vi "Experiment header-Save_Load mov cor section.vi"(7 "Input Mode (ref)":enum16{"Use reference", "Use folder path"}(ring), 8 "error in (no error)":errorcluster, 9 "Function":enum16{"Write", "Read"}(ring), 10 "Experiment folder path":path, 11 "Exp header file ref in":T1) -> (0 "error out":errorcluster, 2 "MovCor enabled (value from header file)":bool, 3 "Exp header file ref":T1)   [LabVIEW 2017]
uses:
  <vilib>/Utility/config.llb/Config Data RefNum.ctl
  Global Variables/General Globals.vi
  <vilib>/Utility/config.llb/Read Key (Boolean).vi
  Movement Correction/Globals/gl_Movement correction globals.vi
  <vilib>/Utility/config.llb/Write Key (Boolean).vi
  <vilib>/Utility/config.llb/Write Key (String).vi
  <vilib>/Utility/config.llb/NI_LVConfig.lvlib
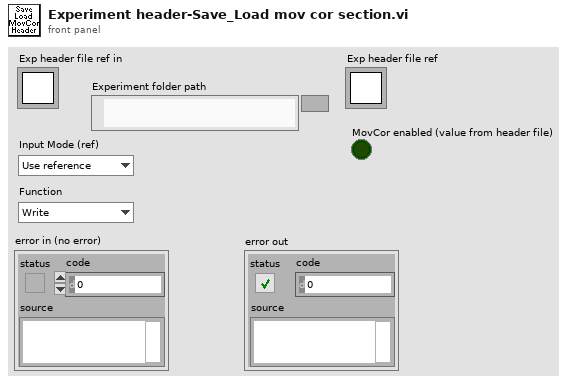
[diagram p1: front panel]
types:
  T1 = typedef "NI_LVConfig.lvlib/Config Data RefNum.ctl" = refnum<k1>
  T2 = typedef "Fixed strings.ctl" = cluster{"ROI file name":string, "Normalised ROI file name":string, "Zplane Pockels values file name":string, "Functional data folder name":string, "Experiment Header file name":string, "Z-stack images folder name":string, "Groups setup rel. path":string, "Groups text file rel. path":string, "TDMS files folder name (F.img)":string, "TDMS files folder name (V.acq)":string, "TDMS files folder name (Pl.acq)":string, "Cycle rel times sequence file":string, "Dynamically called VIs folder name":string, "Time Series folder base name":string}
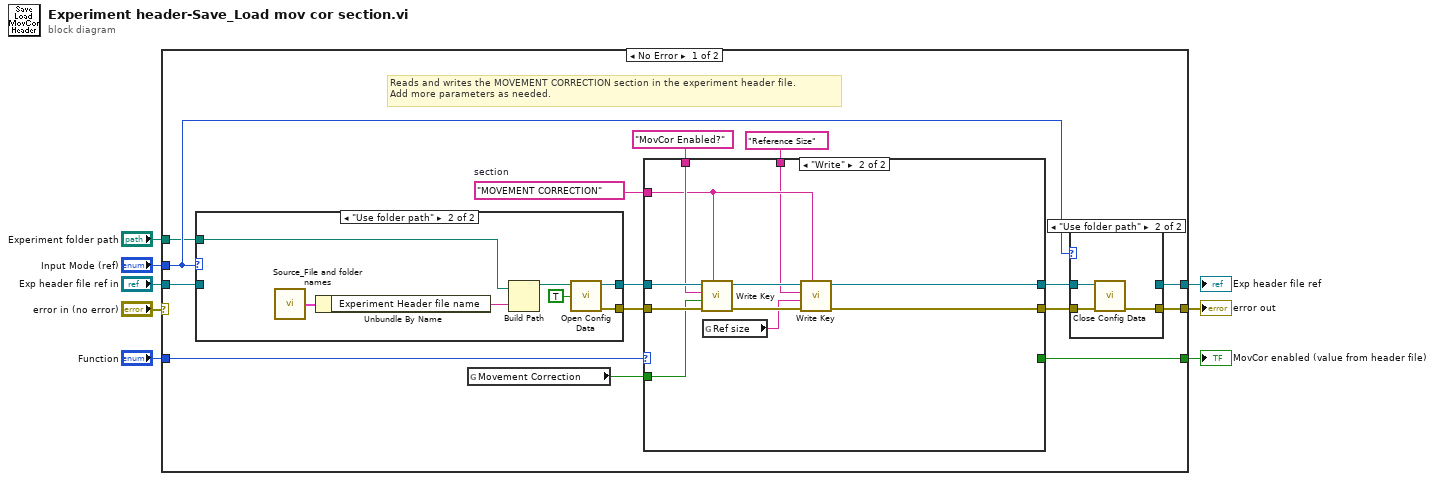
[diagram p0: block diagram]
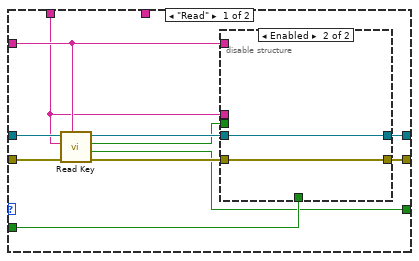
[diagram p4: hidden frame]
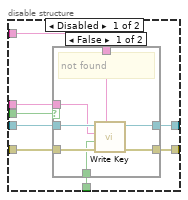
[diagram p5: hidden frame]
diagram:
  n1 = case shown="No Error" "error in (no error)" {
    selector: "error in (no error)" -> [_ w79]
    tunnel: [w17 w79] -> w8
    tunnel: "Function" -> [w16 _]
    tunnel: "Exp header file ref in" -> [w15 w78]
    tunnel: "Input Mode (ref)" -> [w14 _]
    tunnel: [w13 w78] -> w3
    tunnel: [w11 _] -> w2
    tunnel: "Experiment folder path" -> [w10 _]
    frame No Error {
      w22 = "MOVEMENT CORRECTION"  # section
      # "Reads and writes the MOVEMENT CORRECTION section in the experiment header file.\nAdd more parameters as needed."
      n2 = case shown="\"Use folder path\"" w14 {
        tunnel: [_ w36] -> w21
        tunnel: [w29 w35] -> w18
        tunnel: w15 -> [w29 _]
        tunnel: w10 -> [_ w30]
        frame "Use reference", Default {
        }
        frame "Use folder path" {
          n3 = call "Source_File and folder names.vi"() -> ("Fixed strings"=w31:T2)  [unwired: 1 in]
          n4 = Unbundle By Name(w31) -> ("Experiment Header file name"=w32:string)
          n5 = Build Path(base path=w30, name or relative path=w32) -> (appended path=w33:path)
          n6 = call <vilib>:"Open Config Data.vi"("create file if necessary (T)"=TRUE, "configuration file path"=w33) -> ("error out"=w36:errorcluster, "refnum"=w35:T1)  [unwired: 7 in, 1 out]
        }
      }
      n7 = global read "General Globals.vi" "Movement Correction"() -> (w12:bool)
      n8 = case shown="\"Write\"" w16 {
        tunnel: w18 -> [w47 w77]
        tunnel: [w43 w71] -> w19
        tunnel: [w42 w70] -> w20
        tunnel: w21 -> [w46 w76]
        tunnel: w22 -> [w41 w69]
        tunnel: "MovCor Enabled?" ("key") -> [w40 w75]
        tunnel: w12 -> [w39 w74]
        tunnel: [w37 _] -> w11
        tunnel: "Reference Size" ("section") -> [_ w68]
        frame "Read" {
          n9 = call-poly <vilib>:"Read Key.vi"("section"=w41, "error in (no error)"=w46, "key"=w40, "refnum"=w47) -> ("error out"=w44:errorcluster, "value"=w37:bool, "found?"=w38:bool, "refnum out"=w45:T1)  [unwired: 4 in]
          n10 = disable-structure shown="Enabled" {
            disable-tunnel: w45 -> [w55 w66]
            disable-tunnel: w44 -> [w54 w65]
            disable-tunnel: [w53 w66] -> w43
            disable-tunnel: [w52 w65] -> w42
            disable-tunnel: w41 -> [w51 _]
            disable-tunnel: w40 -> [w50 _]
            disable-tunnel: w39 -> [w49 _]
            disable-tunnel: w38 -> [w48 _]
            frame Disabled {
              n11 = case shown="False" w48 {
                tunnel: w55 -> [w62 w64]
                tunnel: w54 -> [w61 w63]
                tunnel: [w60 w64] -> w53
                tunnel: [w59 w63] -> w52
                tunnel: w51 -> [w58 _]
                tunnel: w50 -> [w57 _]
                tunnel: w49 -> [w56 _]
                frame False {
                  # "not found"
                  n12 = call-poly <vilib>:"Write Key.vi"("section"=w58, "error in (no error)"=w61, "value"=w56, "key"=w57, "refnum"=w62) -> ("error out"=w59:errorcluster, "refnum out"=w60:T1)  [unwired: 4 in, 1 out]
                }
                frame True {
                  # "found"
                }
              }
            }
            frame Enabled {
            }
          }
        }
        frame "Write" {
          n13 = call-poly <vilib>:"Write Key.vi"("section"=w69, "error in (no error)"=w76, "value"=w74, "key"=w75, "refnum"=w77) -> ("error out"=w72:errorcluster, "refnum out"=w73:T1)  [unwired: 4 in, 1 out]
          n14 = global read "gl_Movement correction globals.vi" "Ref size"() -> (w67:string)
          n15 = call-poly <vilib>:"Write Key.vi"("section"=w69, "error in (no error)"=w72, "value"=w67, "key"=w68, "refnum"=w73) -> ("error out"=w70:errorcluster, "refnum out"=w71:T1)  [unwired: 4 in, 1 out]
        }
      }
      n16 = case shown="\"Use folder path\"" w14 {
        tunnel: w20 -> [w24 w28]
        tunnel: w19 -> [w25 w27]
        tunnel: [w24 w26] -> w17
        tunnel: [w25 _] -> w13
        frame "Use reference", Default {
        }
        frame "Use folder path" {
          n17 = call <vilib>:"Close Config Data.vi"("error in (no error)"=w28, "refnum"=w27) -> ("error out"=w26:errorcluster)  [unwired: 8 in, 1 out]
        }
      }
    }
    frame Error {
    }
  }
  "error out" <- w8
  "Exp header file ref" <- w3
  "MovCor enabled (value from header file)" <- w2
